vi "ROE200_Move.vi"(6 "error in (no error)":errorcluster, 7 "VISA resource name 2":refnum<visa-resource-name>, 8 "Z":u32, 9 "Y":u32, 10 "X":u32) -> (4 "error out":errorcluster, 5 "VISA resource name out":refnum<visa-resource-name>)   [LabVIEW 2019]
panel:
  out "concatenated string":string
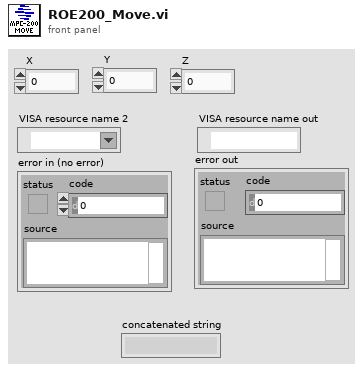
[diagram p1: front panel]
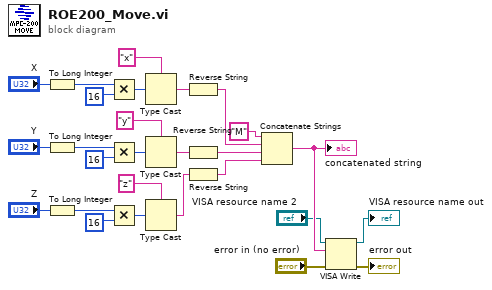
[diagram p0: block diagram]
diagram:
  n1 = To Long Integer(number="X") -> (32bit integer=w5:i32)
  n2 = To Long Integer(number="Y") -> (32bit integer=w1:i32)
  n3 = To Long Integer(number="Z") -> (32bit integer=w3:i32)
  n4 = Multiply(x=w5, y=16) -> (x*y=w26:i32)
  n5 = Multiply(x=w1, y=16) -> (x*y=w23:i32)
  n6 = Multiply(x=w3, y=16) -> (x*y=w20:i32)
  n7 = Type Cast(type="x", x=w26) -> (*(type *) &x=w17:string)
  n8 = Type Cast(type="y", x=w23) -> (*(type *) &x=w15:string)
  n9 = Type Cast(type="z", x=w20) -> (*(type *) &x=w16:string)
  n10 = Reverse String(1:w17) -> (0:w12:string)
  n11 = Reverse String(1:w15) -> (0:w14:string)
  n12 = Reverse String(1:w16) -> (0:w13:string)
  n13 = Concatenate Strings("M", w12, w14, w13) -> (w11:string)
  "concatenated string" <- w11
  n14 = VISA Write(VISA resource name="VISA resource name 2", write buffer=w11, error in (no error)="error in (no error)") -> (VISA resource name out=→"VISA resource name out":refnum<visa-resource-name>, error out=→"error out":errorcluster)  [unwired: 1 out]
